vi "Register Channel.vi"(8 "error in (no error)":errorcluster, 9 "Channel":refnum<class "CIFChannels.lvclass">, 11 "CIFChannelMng in":refnum<class "CIFChannelMng.lvclass">) -> (0 "error out":errorcluster, 3 "CIFChannelMng out":refnum<class "CIFChannelMng.lvclass">)   [LabVIEW 2021, in "CIFChannelMng.lvclass"]
uses:
  CIFChannelMng.lvclass
  CIFCore/Common/CIFCoreCommon.lvlib
  CIFCore/Common/Typedef/Errors.ctl
  CIFChannels/CIFChannels.lvclass
  CIFChannels/Typedef/Direction.ctl
  typedef/Channel List for OOB.ctl
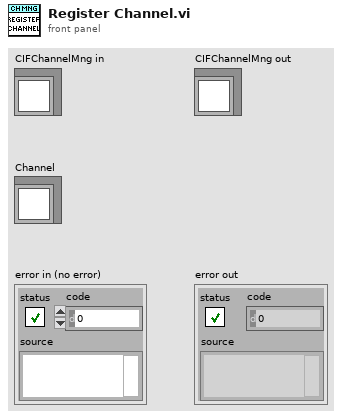
[diagram p1: front panel]
types:
  T1 = typedef "CIFCoreCommon.lvlib/Errors.ctl" = enum16{"Invalid Clock ID", "Long Sleep", "gRPC Server Not Found", "Config Parse", "Timestamp Wrap", "Delayed Execution", "Duplicate Channel", "Missing Channel", "Incorrect Type", "Flatten Error", "Unflatten Data", "Unique Name", "Plugin Not Found"}
  T2 = typedef "CIFChannels.lvclass/Direction.ctl" = enum16{"Publisher", "Subscriber"}
  T3 = typedef "CIFChannelMng.lvclass/Channel List for OOB.ctl" = cluster{"Name":string, "Direction":T2, "Type":string, "Connected?":bool, "Connected Name":string, "Custom Config Data":u8[], "Forced?":bool}
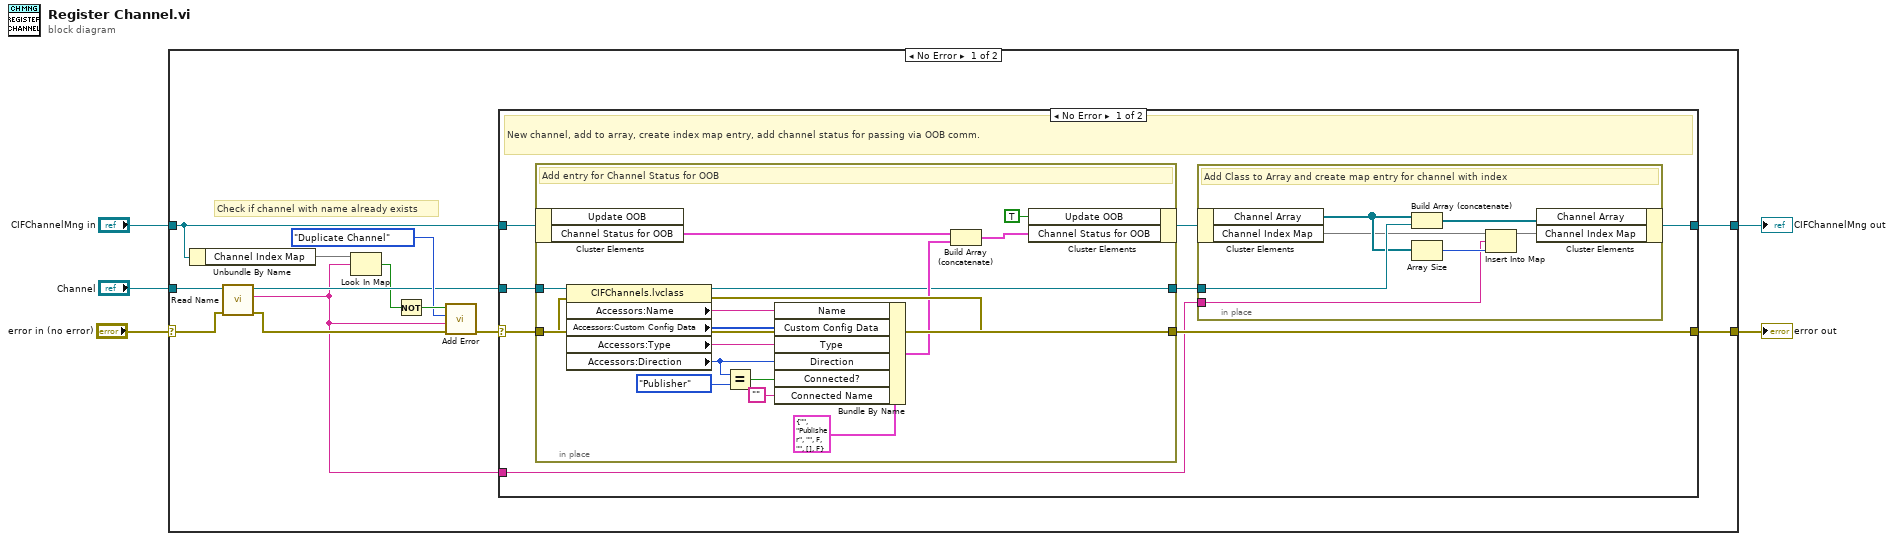
[diagram p0: block diagram]
diagram:
  n1 = case shown="No Error" "error in (no error)" {
    selector: "error in (no error)" -> [w14 w52]
    tunnel: [w13 w52] -> w4
    tunnel: [w11 w51] -> w2
    tunnel: "CIFChannelMng in" -> [w9 w51]
    tunnel: "Channel" -> [w15 _]
    frame No Error {
      # "Check if channel with name already exists"
      n2 = Unbundle By Name(w9) -> ("Channel Index Map"=w8:map{string, i32})
      n3 = call "Read Name.vi"("error in (no error)"=w14, "CIFChannels in"=w15) -> ("error out"=w7:errorcluster, "Name"=w6:string, "CIFChannels out"=w12:refnum<class "CIFChannels.lvclass">)  [unwired: 7 in]
      n4 = Look In Map(map=w8, key=w6) -> (key not found?=w10:bool)  [unwired: 1 in, 1 out]
      n5 = Not(x=w10) -> (.not. x?=w17:bool)
      n6 = call "Add Error.vi"("error in (no error)"=w7, "String to Append"=w6, "Error"=Errors."Duplicate Channel", "Insert Error"=w17) -> ("error out"=w13:errorcluster)  [unwired: 7 in]
      n7 = case shown="No Error" w13 {
        selector: w13 -> [w25 w49]
        tunnel: w9 -> [w23 w50]
        tunnel: w12 -> [w22 _]
        tunnel: [w18 w50] -> w11
        tunnel: [w24 w49] -> _
        tunnel: w6 -> [w19 _]
        frame No Error {
          # "New channel, add to array, create index map entry, add channel status for passing via OOB comm."
          n8 = in-place {
            in-place-border: w22 -> [w48]
            in-place-border: w25 -> [w44]
            in-place-border: [w43] -> w24
            in-place-border: [w33] -> w20
            # "Add entry for Channel Status for OOB"
            n9 = in-place-cluster #1(w23) -> ("Channel Status for OOB"=w36:T3[])  [unwired: 1 out]
            n10 = property class="CIFChannels.lvclass"(reference=w48, error in=w44) -> (reference out=w33:refnum<class "CIFChannels.lvclass">, error out=w43:errorcluster, "Accessors:Name"=w38:string, "Accessors:Custom Config Data"=w45:u8[], "Accessors:Type"=w46:string, "Accessors:Direction"=w41:T2)
            n11 = Equal?(x=w41, y=Direction."Publisher") -> (x = y?=w39:bool)
            n12 = Bundle By Name(cluster=T3 {"Name"="", "Direction"=enum."Publisher", "Type"="", "Connected?"=FALSE, "Connected Name"="", "Custom Config Data"=[], "Forced?"=FALSE} ("Channel List"), "Name"=w38, "Custom Config Data"=w45, "Type"=w46, "Direction"=w41, "Connected?"=w39, "Connected Name"="") -> (w37:T3)
            n13 = Build Array (concatenate)(w36, w37) -> (w35:T3[])
            n14 = in-place-cluster #1("Update OOB"=TRUE, "Channel Status for OOB"=w35) -> (w21:refnum<class "CIFChannelMng.lvclass">)
          }
          n15 = in-place {
            in-place-border: w20 -> [w32]
            in-place-border: w19 -> [w26]
            # "Add Class to Array and create map entry for channel with index"
            n16 = in-place-cluster #2(w21) -> ("Channel Array"=w30:refnum<class "CIFChannels.lvclass">[], "Channel Index Map"=w29:map{string, i32})
            n17 = Build Array (concatenate)(w30, w32) -> (w31:refnum<class "CIFChannels.lvclass">[])
            n18 = Array Size(array=w30) -> (size(s)=w27:i32)
            n19 = Insert Into Map(map in=w29, key=w26, value=w27) -> (map out=w28:map{string, i32})  [unwired: 2 out]
            n20 = in-place-cluster #2("Channel Array"=w31, "Channel Index Map"=w28) -> (w18:refnum<class "CIFChannelMng.lvclass">)
          }
        }
        frame Error {
        }
      }
    }
    frame Error {
    }
  }
  "error out" <- w4
  "CIFChannelMng out" <- w2
